vi "SwapInstanceVIUnusedName2 68.vi"(6 "Bindata & descr in":T1, 7 "type":csg, 8 "error in (no error)":errorcluster, 9 "dims":u8=3 min=1 max=3, 11 "kwarg_name":string="testarg") -> (0 "error out":errorcluster, 1 "Array 3D":csg[][][](array[numeric]) format="%.2f", 2 "Array 2D":csg[][](array[numeric]) format="%.2f", 3 "Array 1D":csg[](array[numeric]) format="%.2f", 4 "Bindata & descr out":T1, 5 "bindata":u8[](array[numeric]))   [LabVIEW 2018]
uses:
  Bindata&description.ctl
  Bindata description.ctl
  0ec67612-8c86-4dd9-b2f9-dc84b2183d14.vi
  edabb94f-ff4d-4e9b-981a-31c21108eeaa.vi
  5a682131-a1fc-4e5a-84ee-8d96e1a90371.vi
  c94e0c1e-f66f-489d-8336-9db841bff071.vi
  edabb94f-ff4d-4e9b-981a-31c21108eeaa.vi/9bd72aa4-846e-40e8-b33d-1f7f5b0bb6f2.vi
  5a682131-a1fc-4e5a-84ee-8d96e1a90371.vi/32d487f6-8df3-4d79-81a2-d35d8a1c854a.vi
  c94e0c1e-f66f-489d-8336-9db841bff071.vi/639da369-9e51-445b-9ea7-6ce45e4def21.vi
  edabb94f-ff4d-4e9b-981a-31c21108eeaa.vi/9bd72aa4-846e-40e8-b33d-1f7f5b0bb6f2.vi/37c16e41-d2ac-4b4a-8dd4-ca0c3b647f5b.vi
  5a682131-a1fc-4e5a-84ee-8d96e1a90371.vi/32d487f6-8df3-4d79-81a2-d35d8a1c854a.vi/fb55c8f2-0e0a-435a-855d-f3f6d9692d6e.vi
  c94e0c1e-f66f-489d-8336-9db841bff071.vi/639da369-9e51-445b-9ea7-6ce45e4def21.vi/ce71436f-f8a1-4523-889c-0c346e11518b.vi
  edabb94f-ff4d-4e9b-981a-31c21108eeaa.vi/9bd72aa4-846e-40e8-b33d-1f7f5b0bb6f2.vi/37c16e41-d2ac-4b4a-8dd4-ca0c3b647f5b.vi/df7122e7-354a-4d10-b547-f17d277d1c27.vi
  5a682131-a1fc-4e5a-84ee-8d96e1a90371.vi/32d487f6-8df3-4d79-81a2-d35d8a1c854a.vi/fb55c8f2-0e0a-435a-855d-f3f6d9692d6e.vi/176fb102-2398-47ce-aecd-749389df5fd3.vi
  c94e0c1e-f66f-489d-8336-9db841bff071.vi/639da369-9e51-445b-9ea7-6ce45e4def21.vi/ce71436f-f8a1-4523-889c-0c346e11518b.vi/e14b1af1-4b06-4321-ad80-1d0bcc1c194d.vi
  check ID validity.vi
  LV-Julia_ZMQ-Roundtrip_lib.lvlib
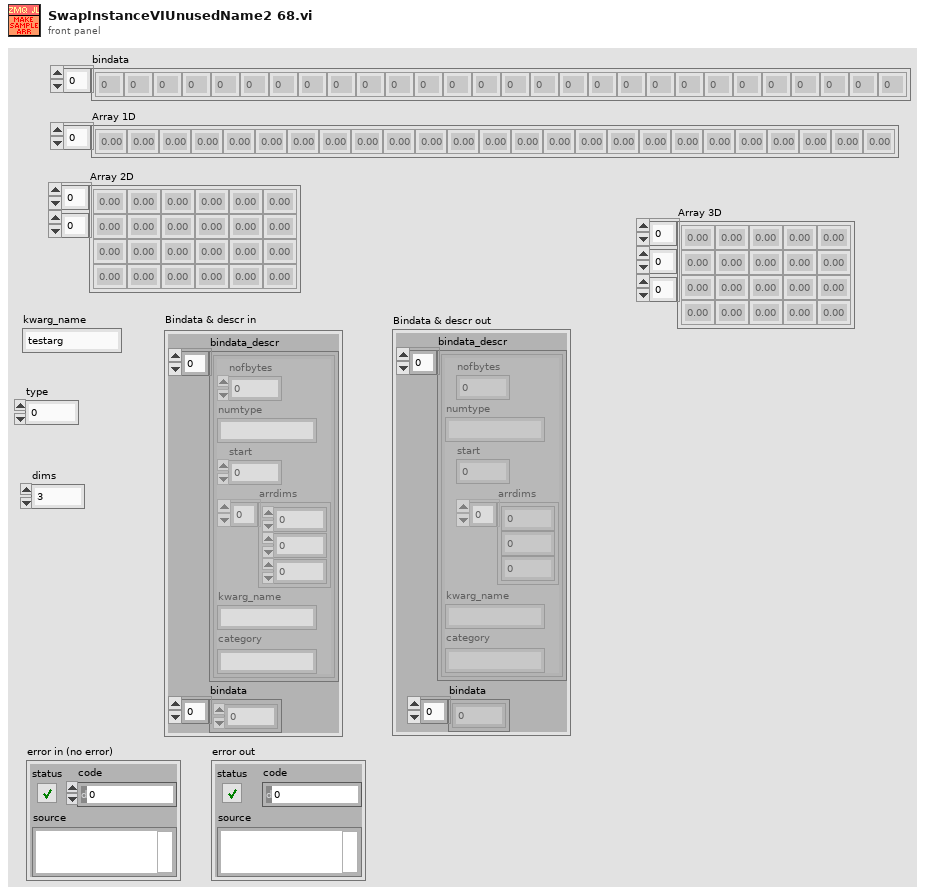
[diagram p1: front panel]
types:
  T1 = typedef "Bindata&description.ctl" = cluster{"bindata_descr":T2[], "bindata":u8[]}
  T2 = typedef "LV-Julia_ZMQ-Roundtrip_lib.lvlib/Bindata description.ctl" = cluster{"nofbytes":i32, "numtype":string, "start":i32, "arrdims":i32[], "kwarg_name":string, "category":string}
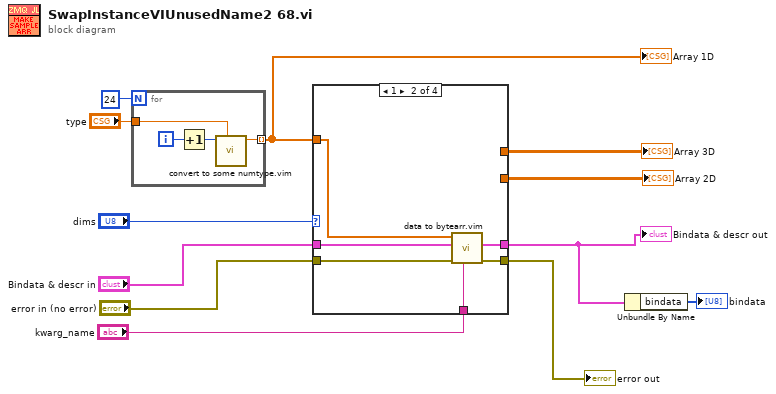
[diagram p0: block diagram]
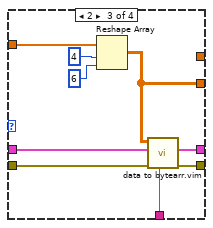
[diagram p3: hidden frame]
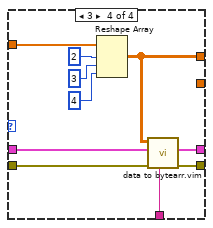
[diagram p4: hidden frame]
diagram:
  n1 = for {
    N: 24 -> [_]
    tunnel: [w14] -> w11 mode=indexing
    tunnel: "type" -> [w13]
    i -> [w16]
    n2 = Increment(x=w16) -> (x+1=w15:i32)
    n3 = call "convert to some numtype.vim"("type"=w13, "Numeric in"=w15) -> ("Numeric out"=w14:csg)  [unwired: 9 in]
  }
  "Array 1D" <- w11
  n4 = case shown="1" "dims" {
    tunnel: [_ _ _ w42] -> w12
    tunnel: w11 -> [_ w23 w30 w38]
    tunnel: "kwarg_name" -> [_ w22 w29 w37]
    tunnel: "error in (no error)" -> [w17 w21 w28 w36]
    tunnel: [w17 w20 w27 w35] -> w5
    tunnel: [_ w19 w26 w34] -> w2
    tunnel: [_ _ w25 _] -> w4
    tunnel: "Bindata & descr in" -> [_ w18 w24 w33]
    frame 0, Default {
    }
    frame 1 {
      n5 = call "data to bytearr.vim"("kwarg_name"=w22, "error in (no error)"=w21, "Bindata & descr in"=w18, "data in"=w23) -> ("error out"=w20:errorcluster, "Bindata & descr out"=w19:T1)  [unwired: 5 in, 1 out]
    }
    frame 2 {
      n6 = Reshape Array(w30, 4 ("dimension size"), 6 ("dimension size")) -> (w25:csg[][])
      n7 = call "data to bytearr.vim"("kwarg_name"=w29, "error in (no error)"=w28, "Bindata & descr in"=w24, "data in"=w25) -> ("error out"=w27:errorcluster, "Bindata & descr out"=w26:T1)  [unwired: 5 in, 1 out]
    }
    frame 3 {
      n8 = Reshape Array(w38, 2 ("dimension size"), 3 ("dimension size"), 4 ("dimension size")) -> (w42:csg[][][])
      n9 = call "data to bytearr.vim"("kwarg_name"=w37, "error in (no error)"=w36, "Bindata & descr in"=w33, "data in"=w42) -> ("error out"=w35:errorcluster, "Bindata & descr out"=w34:T1)  [unwired: 5 in, 1 out]
    }
  }
  "Array 3D" <- w12
  "Bindata & descr out" <- w2
  "error out" <- w5
  "Array 2D" <- w4
  n10 = Unbundle By Name(w2) -> ("bindata"=→"bindata":u8[])
